vi "Lifter Pre-Fudge.vi"(1 "Custom Speed":dbl) -> (0 "In Position":bool)   [LabVIEW 2012]
uses:
  Robot Global Data.vi
panel:
  in  "Limits":cluster{"Upper":dbl, "Lower":dbl}={"Upper"=3.62, "Lower"=2.5}
  in  "Custom Position":dbl
  in  "Joystick Mult":dbl=0.5
  out "Pot Voltage":dbl
  in  "Tolerance":dbl=0.01
  in  "Position Voltages":dbl[](array[numeric])=[2.5, 3.42, 3.48, 0.7, 0.7]
  in  "Motor Gain":dbl=15.0
  # "0 - Climb\n1 - Load\n2 - Pre-climb\n3 - Shoot\n4 - Joystick"
  # "0 - Climb"
  # "2.5"
  # "1 - Load"
  # "3.42"
  # "3.48"
  # "2 - Start"
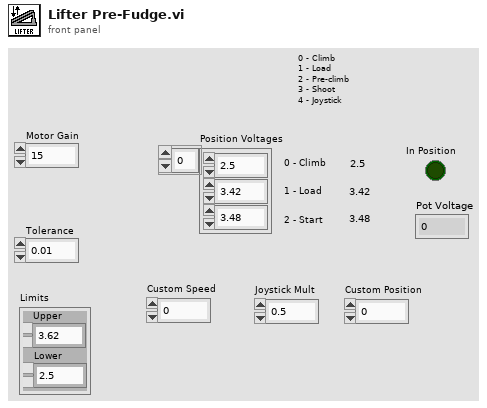
[diagram p1: front panel]
types:
  T1 = typedef "WPI_AnalogChannelDevRef.ctl" = cluster{"DevStatus":errorcluster, "Analog Module":T2, "Analog Channel":T3}
  T2 = typedef "FPGA_TypedefAnalogModule.ctl" = enum16{"Analog Module 1", "Analog Module 2"}
  T3 = typedef "FPGA_AIChannel.ctl" = enum8{"AI 1", "AI 2", "AI 3", "AI 4", "AI 5", "AI 6", "AI 7", "AI 8", "Invalid"}
  T4 = typedef "WPI_MotorControlDeviceRef.ctl" = cluster{"DeviceStatus":errorcluster, "Type":enum16{"PWM", "CAN"}, "PWM":cluster{"Digital Module":T5, "PWM Channel":T6, "DeadBand":T7}, "CAN":cluster{"Device Number":u8, "Control Mode":T8, "Semaphore":T9, "Max Vout":dbl}, "Invert":bool, "TransformRef":T10, "InvTransformRef":T10}
  T5 = typedef "FPGA_TypedefDigitalModule.ctl" = enum16{"Digital Module 1", "Digital Module 2"}
  T6 = typedef "FPGA_DIOPWMChannel.ctl" = enum8{"PWM 1", "PWM 2", "PWM 3", "PWM 4", "PWM 5", "PWM 6", "PWM 7", "PWM 8", "PWM 9", "PWM 10", "Invalid"}
  T7 = typedef "WPI_PWMDeadband.ctl" = cluster{"Name":string, "maxPositivePwm":i32, "minPositivePwm":i32, "centerPwm":i32, "maxNegativePwm":i32, "minNegativePwm":i32, "angularRange":u16}
  T8 = typedef "WPI_CANJaguar_ControlMode.ctl" = enum8{"Percent VBus", "Current", "Speed", "Position", "Voltage"}
  T9 = typedef "Semaphore RefNum" = refnum<k1>
  T10 = typedef "WPI_PWMTransform_ConPane.ctl" = refnum<vi>
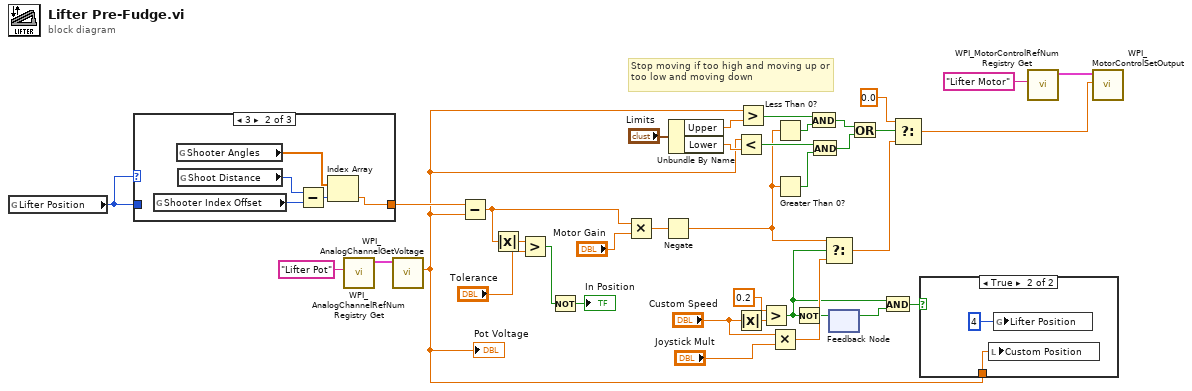
[diagram p0: block diagram]
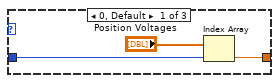
[diagram p2: hidden frame]
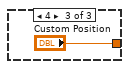
[diagram p3: hidden frame]
diagram:
  # "Stop moving if too high and moving up or too low and moving down"
  n1 = global read "Robot Global Data.vi" "Lifter Position"() -> (w16:i8)
  n2 = case shown="3" w16 {
    tunnel: [w40 w44 "Custom Position"] -> w34
    tunnel: w16 -> [w39 _ _]
    frame 0, Default {
      n3 = Index Array(array="Position Voltages", index=w39) -> (element=w40:dbl)
    }
    frame 3 {
      n4 = global read "Robot Global Data.vi" "Shooter Index Offset"() -> (w41:i32)
      n5 = global read "Robot Global Data.vi" "Shooter Angles"() -> (w45:dbl[])
      n6 = global read "Robot Global Data.vi" "Shoot Distance"() -> (w42:i32)
      n7 = Subtract(x=w42, y=w41) -> (x-y=w43:i32)
      n8 = Index Array(array=w45, index=w43) -> (element=w44:dbl)
    }
    frame 4 {
    }
  }
  n9 = call <vilib>:"WPI_AnalogChannelRefNum Registry Get.vi"("refnum name"="Lifter Pot") -> ("AIDeviceRef"=w37:T1)  [unwired: 9 in, 1 out]
  n10 = call <vilib>:"WPI_AnalogChannelGetVoltage.vi"("AIDeviceRef"=w37) -> ("Voltage"=w3:dbl)  [unwired: 8 in, 2 out]
  "Pot Voltage" <- w3
  n11 = Subtract(x=w34, y=w3) -> (x-y=w30:dbl)
  n12 = Absolute Value(x=w30) -> (abs(x)=w28:dbl)
  n13 = Greater?(x=w28, y="Tolerance") -> (0:w29:bool)
  n14 = Not(x=w29) -> (.not. x?=→"In Position":bool)
  n15 = Multiply(x=w30, y="Motor Gain") -> (x*y=w32:dbl)
  n16 = Negate(x=w32) -> (-x=w1:dbl)
  n17 = Unbundle By Name("Limits") -> ("Upper"=w5:dbl, "Lower"=w4:dbl)
  n18 = Less?(x=w3, y=w4) -> (x < y?=w8:bool)
  n19 = Absolute Value(x="Custom Speed") -> (abs(x)=w19:dbl)
  n20 = Greater?(x=w3, y=w5) -> (0:w11:bool)
  n21 = Greater?(x=0.2, y=w19) -> (0:w18:bool)
  n22 = Multiply(x="Custom Speed", y="Joystick Mult") -> (x*y=w22:dbl)
  n23 = Less Than 0?(x=w1) -> (x < 0?=w2:bool)
  n24 = Greater Than 0?(x=w1) -> (x > 0?=w7:bool)
  n25 = Not(x=w18) -> (.not. x?=w17:bool)
  n26 = And(x=w11, y=w2) -> (x .and. y?=w10:bool)
  n27 = And(x=w8, y=w7) -> (x .and. y?=w9:bool)
  n28 = Select(t=w1, s=w18, f=w22) -> (s? t:f=w15:dbl)
  n29 = feedback-in #1(w17) -> ()
  n30 = feedback #1() -> (w20:bool)  [unwired: 1 in]
  n31 = Or(x=w10, y=w9) -> (x .or. y?=w12:bool)
  n32 = And(x=w18, y=w20) -> (x .and. y?=w21:bool)
  n33 = Select(t=0.0, s=w12, f=w15) -> (s? t:f=w13:dbl)
  n34 = case shown="True" w21 {
    tunnel: w3 -> [_ w48]
    frame False {
    }
    frame True {
      n35 = local write "Custom Position"(w48) -> ()
      n36 = global write "Robot Global Data.vi" "Lifter Position"(i8 4 ("Desired Position")) -> ()
    }
  }
  n37 = call <vilib>:"WPI_MotorControlRefNum Registry Get.vi"("refnum name"="Lifter Motor") -> ("MotorControlDevRef"=w33:T4)  [unwired: 9 in, 1 out]
  n38 = call <vilib>:"WPI_MotorControlSetOutput.vi"("Output"=w13, "MotorControlDevRef"=w33) -> ()  [unwired: 7 in, 3 out]
